vi "_098.vi"() -> ()   [LabVIEW 2020]
panel:
  out "size(s)":i32
  out "Array":i32[](array[numeric])
  # "What will be the value of size(s) after the code completes execution?"
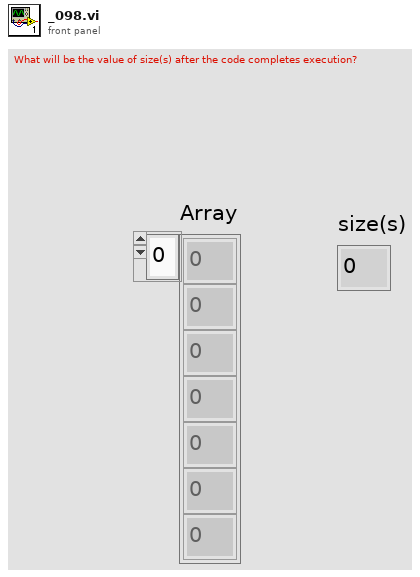
[diagram p1: front panel]
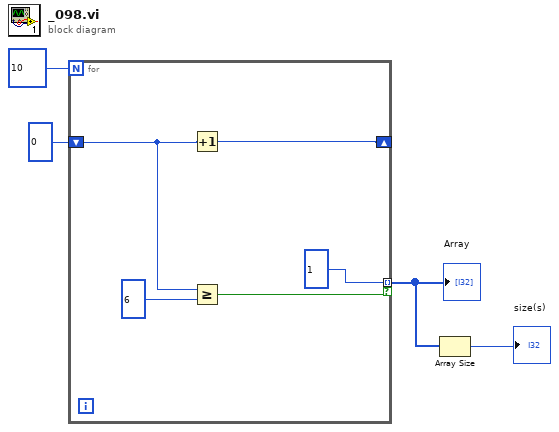
[diagram p0: block diagram]
diagram:
  n1 = for {
    N: 10 -> [_]
    tunnel: [1] -> w3 mode=indexing if=w7
    shift-right: [w6] -> _
    shift-left: 0 -> [w5]
    n2 = Increment(x=w5) -> (x+1=w6:i32)
    n3 = Greater Or Equal?(x=w5, y=6) -> (x >= y?=w7:bool)
  }
  "Array" <- w3
  n4 = Array Size(array=w3) -> (size(s)=→"size(s)":i32)
